vi "GetStateData.vi"(11 "Pod in":T18={"DriveMotorRef"={"DeviceStatus"={"status"=FALSE, "code"=0, "source"=""}, "Type"=enum."PWM", "PWM"={"Controller"=enum."Controller 1", "PWM Channel"=enum."Invalid", "DeadBand"={"Name"="", "maxPositivePwm"=0, "minPositivePwm"=0, "centerPwm"=0, "maxNegativePwm"=0, "minNegativePwm"=0, "angularRange"=0}}, "CAN"={"Device Number"=0, "Control Mode"=enum."Percent VBus", "Semaphore"=refnum, "Max Vout"=12.0, "TalonSRX Control Mode"=enum."Percent VBus"}, "Invert"=FALSE, "TransformRef"=refnum, "InvTransformRef"=refnum}, "TurretMotorRef"={"DeviceStatus"={"status"=FALSE, "code"=0, "source"=""}, "Type"=enum."PWM", "PWM"={"Controller"=enum."Controller 1", "PWM Channel"=enum."Invalid", "DeadBand"={"Name"="", "maxPositivePwm"=0, "minPositivePwm"=0, "centerPwm"=0, "maxNegativePwm"=0, "minNegativePwm"=0, "angularRange"=0}}, "CAN"={"Device Number"=0, "Control Mode"=enum."Percent VBus", "Semaphore"=refnum, "Max Vout"=12.0, "TalonSRX Control Mode"=enum."Percent VBus"}, "Invert"=FALSE, "TransformRef"=refnum, "InvTransformRef"=refnum}, "Turret Encoder"={"AIDeviceRef"={"DevStatus"={"status"=FALSE, "code"=0, "source"=""}, "Controller"=enum."Controller 1", "Analog Channel"=enum."AI 0"}, "Turret Analog Location"=enum."RoboRio"}, "Drive Encoder"={"EncoderDevRef"={"DevStatus"={"status"=FALSE, "code"=0, "source"=""}, "EncoderIndex"=enum."Invalid", "CounterIndex"=enum."Invalid", "DistancePerCount"=1.0, "Decoding Type"=enum."4x"}, "Drive Encoder Location"=enum."RoboRio"}, "Pod position (RCS)"={"X"=0.0, "Y"=0.0, "Z"=0.0}, "Data"={"Drive Motor Output"=0.0, "Turret Motor Output"=0.0, "Wheel RPM"=0.0, "Turret Angle"=0.0, "Turret angle offset"=0.0, "Transmission moment of inertia"=0.0, "Transmission efficiency"=0.0, "Wheel dist / rev"=0.0, "Turret moment of inertia"=0.0, "Inv. turret encoder"=FALSE, "Inv. drive encoder"=FALSE}}) -> (2 "Pod States":T1, 3 "Pod out":T18={"DriveMotorRef"={"DeviceStatus"={"status"=FALSE, "code"=0, "source"=""}, "Type"=enum."PWM", "PWM"={"Controller"=enum."Controller 1", "PWM Channel"=enum."Invalid", "DeadBand"={"Name"="", "maxPositivePwm"=0, "minPositivePwm"=0, "centerPwm"=0, "maxNegativePwm"=0, "minNegativePwm"=0, "angularRange"=0}}, "CAN"={"Device Number"=0, "Control Mode"=enum."Percent VBus", "Semaphore"=refnum, "Max Vout"=12.0, "TalonSRX Control Mode"=enum."Percent VBus"}, "Invert"=FALSE, "TransformRef"=refnum, "InvTransformRef"=refnum}, "TurretMotorRef"={"DeviceStatus"={"status"=FALSE, "code"=0, "source"=""}, "Type"=enum."PWM", "PWM"={"Controller"=enum."Controller 1", "PWM Channel"=enum."Invalid", "DeadBand"={"Name"="", "maxPositivePwm"=0, "minPositivePwm"=0, "centerPwm"=0, "maxNegativePwm"=0, "minNegativePwm"=0, "angularRange"=0}}, "CAN"={"Device Number"=0, "Control Mode"=enum."Percent VBus", "Semaphore"=refnum, "Max Vout"=12.0, "TalonSRX Control Mode"=enum."Percent VBus"}, "Invert"=FALSE, "TransformRef"=refnum, "InvTransformRef"=refnum}, "Turret Encoder"={"AIDeviceRef"={"DevStatus"={"status"=FALSE, "code"=0, "source"=""}, "Controller"=enum."Controller 1", "Analog Channel"=enum."AI 0"}, "Turret Analog Location"=enum."RoboRio"}, "Drive Encoder"={"EncoderDevRef"={"DevStatus"={"status"=FALSE, "code"=0, "source"=""}, "EncoderIndex"=enum."Invalid", "CounterIndex"=enum."Invalid", "DistancePerCount"=1.0, "Decoding Type"=enum."4x"}, "Drive Encoder Location"=enum."RoboRio"}, "Pod position (RCS)"={"X"=0.0, "Y"=0.0, "Z"=0.0}, "Data"={"Drive Motor Output"=0.0, "Turret Motor Output"=0.0, "Wheel RPM"=0.0, "Turret Angle"=0.0, "Turret angle offset"=0.0, "Transmission moment of inertia"=0.0, "Transmission efficiency"=0.0, "Wheel dist / rev"=0.0, "Turret moment of inertia"=0.0, "Inv. turret encoder"=FALSE, "Inv. drive encoder"=FALSE}})   [LabVIEW 2014]
uses:
  <vilib>/Rock Robotics/WPI/MotorControl/WPI_MotorControlDeviceRef.ctl
  <vilib>/Rock Robotics/WPI/MotorControl/WPI_MotorControlType.ctl
  <vilib>/Rock Robotics/SystemInterfaces/Typedef/FPGA_TypedefDigitalModule.ctl
  <vilib>/Rock Robotics/SystemInterfaces/DIO/FPGA_DIOPWMChannel.ctl
  <vilib>/Rock Robotics/WPI/PWM/WPI_PWMDeadband.ctl
  <vilib>/Rock Robotics/WPI/CAN/Jaguar/SubVIs/WPI_CANJaguar_ControlMode.ctl
  <vilib>/Rock Robotics/WPI/CAN/TalonSRX/WPI_CANTalonSRX_APIControlMode.ctl
  <vilib>/Rock Robotics/WPI/PWM/WPI_PWMTransform_ConPane.ctl
  <vilib>/Rock Robotics/WPI/AnalogChannel/WPI_AnalogChannelDevRef.ctl
  <vilib>/Rock Robotics/SystemInterfaces/Typedef/FPGA_TypedefAnalogModule.ctl
  <vilib>/Rock Robotics/SystemInterfaces/AI/FPGA_AIChannel.ctl
  <vilib>/Rock Robotics/WPI/Encoder/WPI_EncoderDevRef.ctl
  <vilib>/Rock Robotics/SystemInterfaces/Encoder/FPGA_EncoderIdx.ctl
  <vilib>/Rock Robotics/SystemInterfaces/Counter/FPGA_CounterCtrSystemIndex.ctl
  <vilib>/Rock Robotics/WPI/Encoder/WPI_EncoderType.ctl
  <vilib>/Rock Robotics/SystemInterfaces/Utilities/FPGA_UtilitiesRead LocalTime.vi
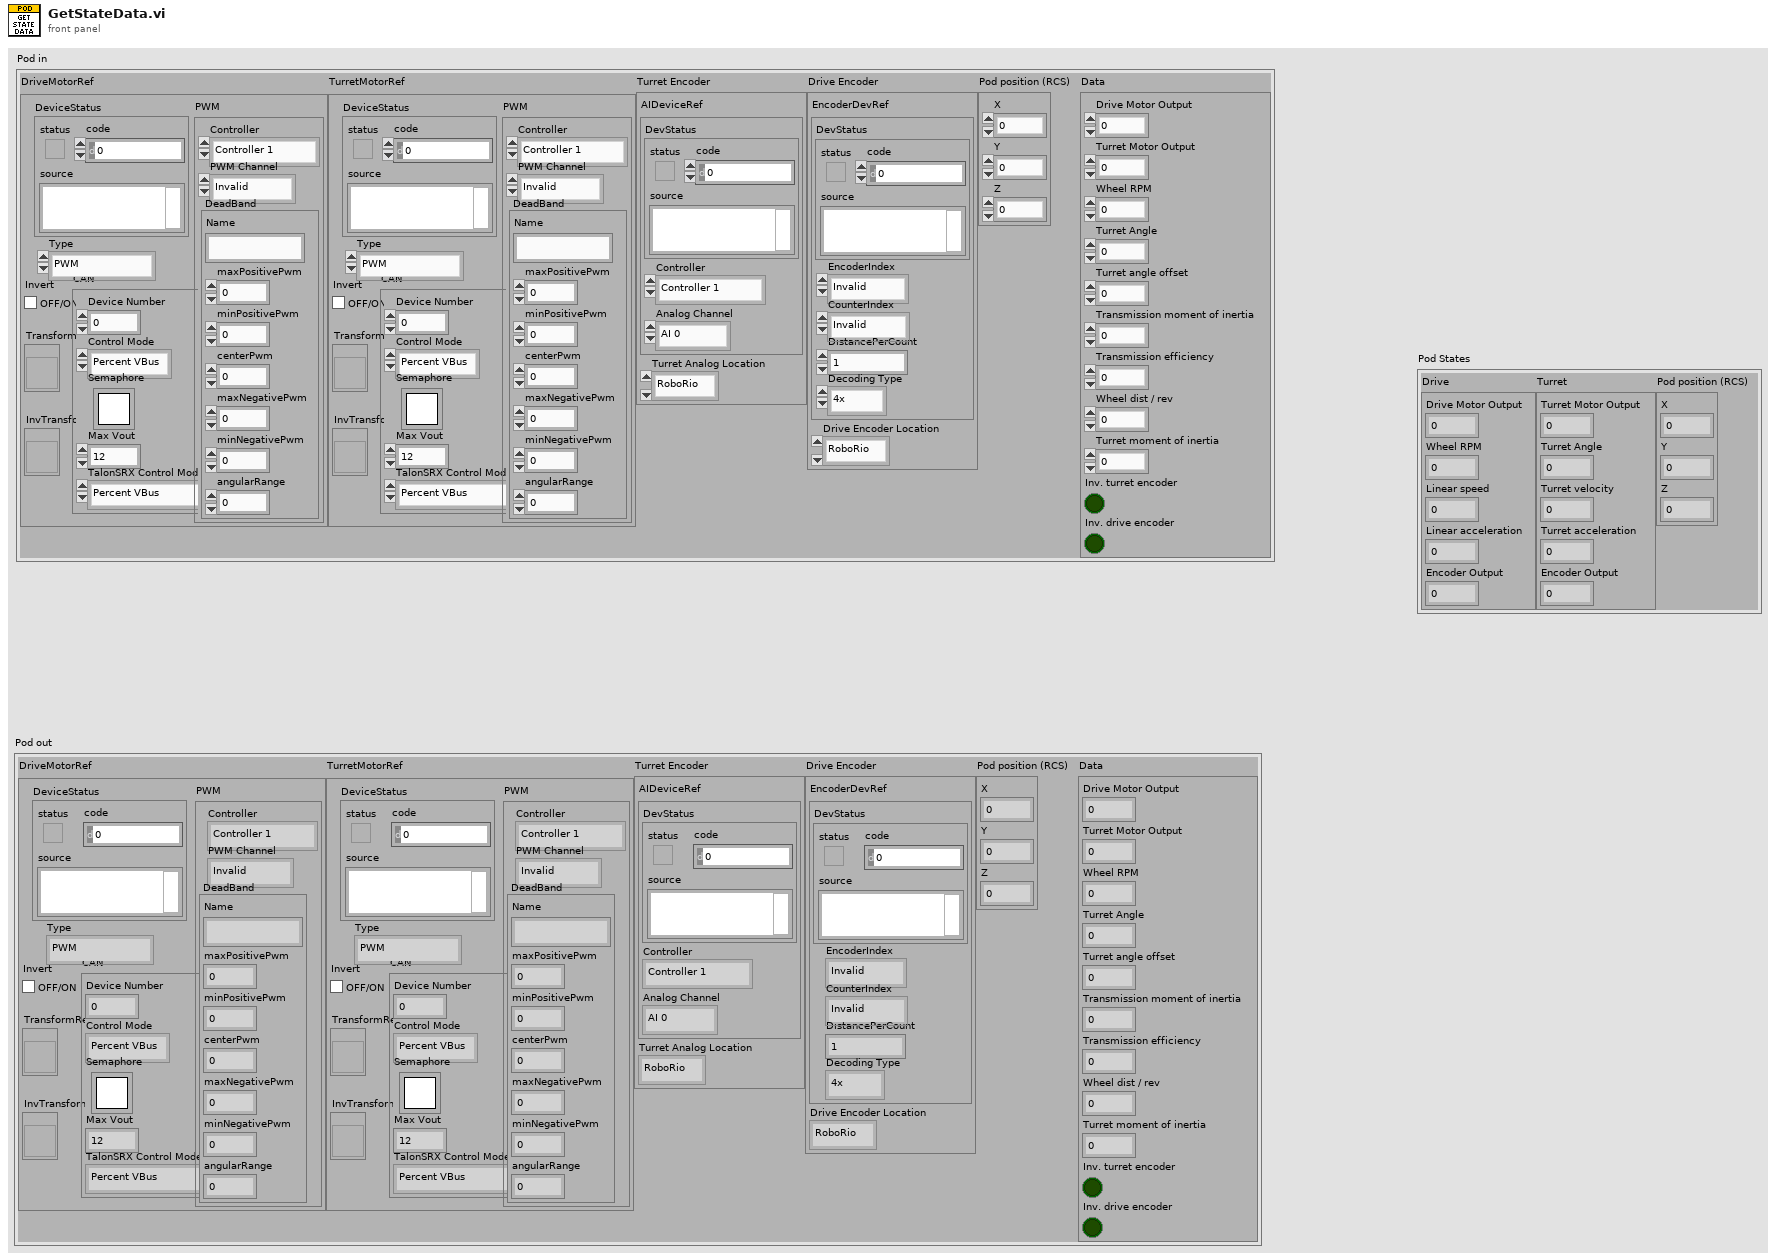
[diagram p1: front panel]
types:
  T1 = cluster{"Drive":cluster{"Drive Motor Output":dbl, "Wheel RPM":dbl, "Linear speed":dbl, "Linear acceleration":dbl, "Encoder Output":dbl}, "Turret":cluster{"Turret Motor Output":dbl, "Turret Angle":dbl, "Turret velocity":dbl, "Turret acceleration":dbl, "Encoder Output":dbl}, "Pod position (RCS)":cluster{"X":dbl, "Y":dbl, "Z":dbl}}
  T2 = typedef "WPI_MotorControlDeviceRef.ctl" = cluster{"DeviceStatus":errorcluster, "Type":T3, "PWM":cluster{"Controller":T4, "PWM Channel":T5, "DeadBand":T6}, "CAN":cluster{"Device Number":u8, "Control Mode":T7, "Semaphore":T8, "Max Vout":dbl, "TalonSRX Control Mode":T9}, "Invert":bool, "TransformRef":T10, "InvTransformRef":T10}
  T3 = typedef "WPI_MotorControlType.ctl" = enum16{"PWM", "CAN", "CANTalonSRX"}
  T4 = typedef "FPGA_TypedefDigitalModule.ctl" = enum16{"Controller 1"}
  T5 = typedef "FPGA_DIOPWMChannel.ctl" = enum8{"PWM 0", "PWM 1", "PWM 2", "PWM 3", "PWM 4", "PWM 5", "PWM 6", "PWM 7", "PWM 8", "PWM 9", "PWM MXP 0", "PWM MXP 1", "PWM MXP 2", "PWM MXP 3", "PWM MXP 4", "PWM MXP 5", "PWM MXP 6", "PWM MXP 7", "PWM MXP 8", "PWM MXP 9", "Invalid"}
  T6 = typedef "WPI_PWMDeadband.ctl" = cluster{"Name":string, "maxPositivePwm":i32, "minPositivePwm":i32, "centerPwm":i32, "maxNegativePwm":i32, "minNegativePwm":i32, "angularRange":u16}
  T7 = typedef "WPI_CANJaguar_ControlMode.ctl" = enum8{"Percent VBus", "Current", "Speed", "Position", "Voltage"}
  T8 = typedef "Semaphore RefNum" = refnum<k1>
  T9 = typedef "WPI_CANTalonSRX_APIControlMode.ctl" = enum8{"Percent VBus", "Speed", "Position", "Slave", "Unchanged / Invalid"}
  T10 = typedef "WPI_PWMTransform_ConPane.ctl" = refnum<vi>
  T11 = typedef "WPI_AnalogChannelDevRef.ctl" = cluster{"DevStatus":errorcluster, "Controller":T12, "Analog Channel":T13}
  T12 = typedef "FPGA_TypedefAnalogModule.ctl" = enum16{"Controller 1"}
  T13 = typedef "FPGA_AIChannel.ctl" = enum8{"AI 0", "AI 1", "AI 2", "AI 3", "AI MXP 0", "AI MXP 1", "AI MXP 2", "AI MXP 3", "Invalid"}
  T14 = typedef "WPI_EncoderDevRef.ctl" = cluster{"DevStatus":errorcluster, "EncoderIndex":T15, "CounterIndex":T16, "DistancePerCount":dbl, "Decoding Type":T17}
  T15 = typedef "FPGA_EncoderIdx.ctl" = enum8{"Enc 0", "Enc 1", "Enc 2", "Enc 3", "Enc 4", "Enc 5", "Enc 6", "Enc 7", "Invalid"}
  T16 = typedef "FPGA_CounterCtrSystemIndex.ctl" = enum8{"Ctr 0", "Ctr 1", "Ctr 2", "Ctr 3", "Ctr 4", "Ctr 5", "Ctr 6", "Ctr 7", "Invalid"}
  T17 = typedef "WPI_EncoderType.ctl" = enum16{"1x", "2x", "4x"}
  T18 = cluster{"DriveMotorRef":T2, "TurretMotorRef":T2, "Turret Encoder":cluster{"AIDeviceRef":T11, "Turret Analog Location":enum16{"RoboRio", "Drive SRX", "Turret SRX"}}, "Drive Encoder":cluster{"EncoderDevRef":T14, "Drive Encoder Location":enum16{"RoboRio", "Drive SRX", "Turret SRX"}}, "Pod position (RCS)":cluster{"X":dbl, "Y":dbl, "Z":dbl}, "Data":cluster{"Drive Motor Output":dbl, "Turret Motor Output":dbl, "Wheel RPM":dbl, "Turret Angle":dbl, "Turret angle offset":dbl, "Transmission moment of inertia":dbl, "Transmission efficiency":dbl, "Wheel dist / rev":dbl, "Turret moment of inertia":dbl, "Inv. turret encoder":bool, "Inv. drive encoder":bool}}
  T19 = typedef "WPI_CANTalonSRX_GlobalStatus.ctl" = cluster{"Applied Throttle":dbl, "Module Enabled":bool, "CAN Error":errorcluster, "Closed Loop Error":dbl, "Forward Limit Switch Closed":bool, "Reverse Limit Switch Closed":bool, "Sensor Position":dbl, "Sensor Velocity":dbl, "Current":dbl, "Sticky Fault - Over Temp":bool, "Sticky Fault - Under Voltage":bool, "Sticky Fault - Forward Limit":bool, "Sticky Fault - Reverse Limit":bool, "Sticky Fault - Forward Soft Limit":bool, "Sticky Fault - Reverse Soft Limit":bool, "Brake is Enabled":bool, "Encoder Position":dbl, "Encoder Velocity":dbl, "Encoder Index Count":dbl, "Encoder A Pin State":bool, "Encoder B Pin State":bool, "Encoder Index Pin State":bool, "Analog In":dbl, "Analog In Velocity":dbl, "Temperature (C)":dbl, "Battery Voltage":dbl}
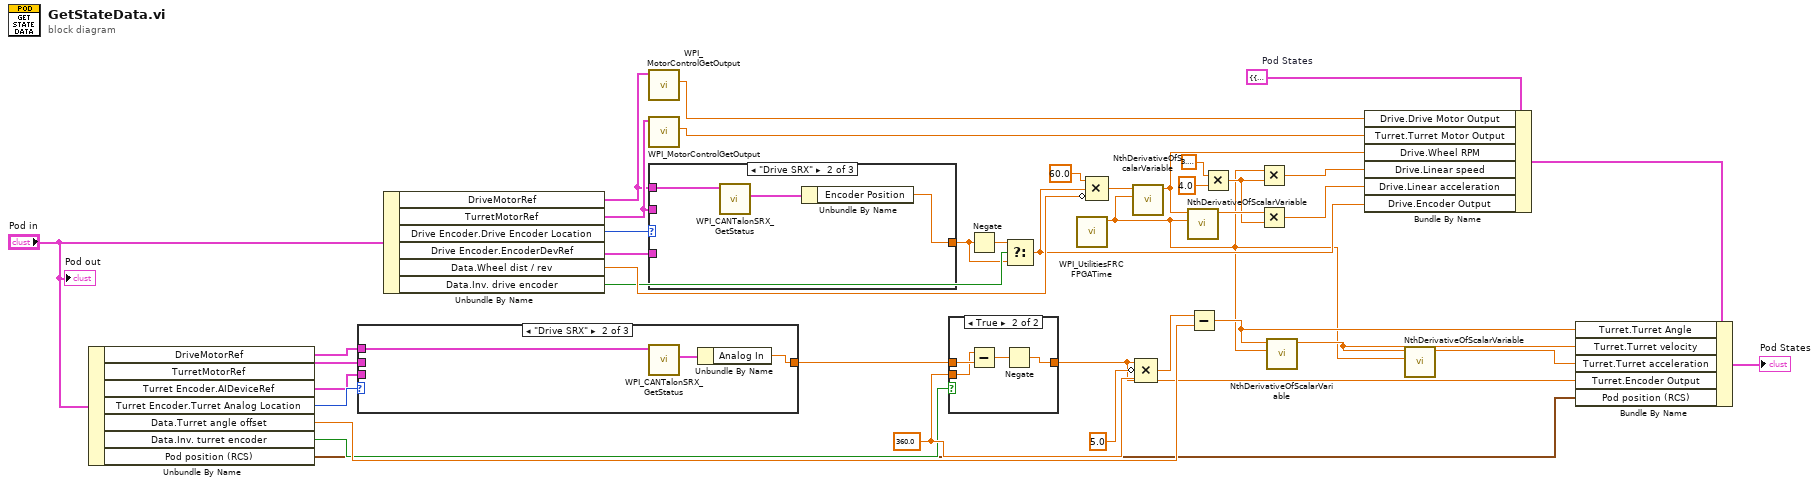
[diagram p0: block diagram]
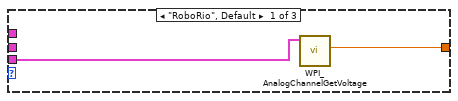
[diagram p3: hidden frame]
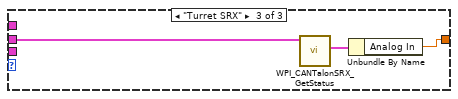
[diagram p4: hidden frame]
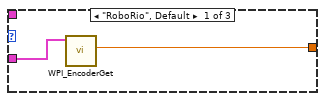
[diagram p5: hidden frame]
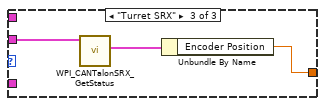
[diagram p6: hidden frame]
diagram:
  w20 = T1 {"Drive"={"Drive Motor Output"=0.0, "Wheel RPM"=0.0, "Linear speed"=0.0, "Linear acceleration"=0.0, "Encoder Output"=0.0}, "Turret"={"Turret Motor Output"=0.0, "Turret Angle"=0.0, "Turret velocity"=0.0, "Turret acceleration"=0.0, "Encoder Output"=0.0}, "Pod position (RCS)"={"X"=0.0, "Y"=0.0, "Z"=0.0}}  # Pod States
  w23 = 360.0 ("value")
  n1 = Unbundle By Name("Pod in") -> ("DriveMotorRef"=w30:T2, "TurretMotorRef"=w31:T2, "Turret Encoder.AIDeviceRef"=w32:T11, "Turret Encoder.Turret Analog Location"=w33:enum16{"RoboRio", "Drive SRX", "Turret SRX"}, "Data.Turret angle offset"=w26:dbl, "Data.Inv. turret encoder"=w22:bool, "Pod position (RCS)"=w12:cluster{"X":dbl, "Y":dbl, "Z":dbl})
  n2 = case shown="\"Drive SRX\"" w33 {
    tunnel: w32 -> [w42 _ _]
    tunnel: w31 -> [_ _ w46]
    tunnel: w30 -> [_ w44 _]
    tunnel: [w41 w43 w47] -> w7
    frame "RoboRio", Default {
      n3 = call <vilib>:"WPI_AnalogChannelGetVoltage.vi"("AIDeviceRef"=w42) -> ("Voltage"=w41:dbl)  [unwired: 8 in, 2 out]
    }
    frame "Drive SRX" {
      n4 = call <vilib>:"WPI_CANTalonSRX_GetStatus.vi"("CAN Talon SRX Ref"=w44) -> ("Talon SRX Status"=w45:T19)  [unwired: 8 in, 2 out]
      n5 = Unbundle By Name(w45) -> ("Analog In"=w43:dbl)
    }
    frame "Turret SRX" {
      n6 = call <vilib>:"WPI_CANTalonSRX_GetStatus.vi"("CAN Talon SRX Ref"=w46) -> ("Talon SRX Status"=w48:T19)  [unwired: 8 in, 2 out]
      n7 = Unbundle By Name(w48) -> ("Analog In"=w47:dbl)
    }
  }
  n8 = Unbundle By Name("Pod in") -> ("DriveMotorRef"=w39:T2, "TurretMotorRef"=w40:T2, "Drive Encoder.Drive Encoder Location"=w38:enum16{"RoboRio", "Drive SRX", "Turret SRX"}, "Drive Encoder.EncoderDevRef"=w37:T14, "Data.Wheel dist / rev"=w36:dbl, "Data.Inv. drive encoder"=w24:bool)
  n9 = call <vilib>:"WPI_MotorControlGetOutput.vi"("MotorControlDevRef"=w39) -> ("Output"=w34:dbl)  [unwired: 8 in, 2 out]
  n10 = call <vilib>:"WPI_MotorControlGetOutput.vi"("MotorControlDevRef"=w40) -> ("Output"=w35:dbl)  [unwired: 8 in, 2 out]
  n11 = case shown="\"Drive SRX\"" w38 {
    tunnel: w40 -> [_ _ w54]
    tunnel: w39 -> [_ w53 _]
    tunnel: w37 -> [w50 _ _]
    tunnel: [w49 w51 w55] -> w10
    frame "RoboRio", Default {
      n12 = call <vilib>:"WPI_EncoderGet.vi"("EncoderDevRef"=w50) -> ("Distance"=w49:dbl)  [unwired: 5 in, 5 out]
    }
    frame "Drive SRX" {
      n13 = call <vilib>:"WPI_CANTalonSRX_GetStatus.vi"("CAN Talon SRX Ref"=w53) -> ("Talon SRX Status"=w52:T19)  [unwired: 8 in, 2 out]
      n14 = Unbundle By Name(w52) -> ("Encoder Position"=w51:dbl)
    }
    frame "Turret SRX" {
      n15 = call <vilib>:"WPI_CANTalonSRX_GetStatus.vi"("CAN Talon SRX Ref"=w54) -> ("Talon SRX Status"=w56:T19)  [unwired: 8 in, 2 out]
      n16 = Unbundle By Name(w56) -> ("Encoder Position"=w55:dbl)
    }
  }
  n17 = case shown="True" w22 {
    tunnel: w7 -> [w57 w61]
    tunnel: w23 -> [_ w60]
    tunnel: [w57 w58] -> w5
    frame False {
    }
    frame True {
      n18 = Subtract(x=w60, y=w61) -> (x-y=w59:dbl)
      n19 = Negate(x=w59) -> (-x=w58:dbl)
    }
  }
  n20 = Negate(x=w10) -> (-x=w25:dbl)
  n21 = Select(t=w25, s=w24, f=w10) -> (s? t:f=w8:dbl)
  n22 = call <vilib>:"WPI_UtilitiesFRC FPGATime.vi"() -> ("FPGA Time"=w1:dbl)  [unwired: 10 in, 1 out]
  n23 = Compound Arithmetic op=MULTIPLY(60.0 ("value"), w8, invert w36) -> (w9:dbl)
  n24 = call "NthDerivativeOfScalarVariable.vi"("FPGA Timestamp"=w1, "X"=w9) -> ("Nth derivative of X"=w11:dbl)  [unwired: 9 in]
  n25 = Compound Arithmetic op=MULTIPLY(w5, invert 5.0 ("value"), w23) -> (w6:dbl)
  n26 = call "NthDerivativeOfScalarVariable.vi"("FPGA Timestamp"=w1, "X"=w11) -> ("Nth derivative of X"=w17:dbl)  [unwired: 9 in]
  n27 = Subtract(x=w6, y=w26) -> (x-y=w4:dbl)
  n28 = Multiply(x=3.141592653589793, y=4.0) -> (x*y=w16:dbl)
  n29 = Multiply(x=w1, y=w16) -> (x*y=w15:dbl)
  n30 = Multiply(x=w17, y=w16) -> (x*y=w14:dbl)
  n31 = call "NthDerivativeOfScalarVariable.vi"("FPGA Timestamp"=w1, "X"=w4) -> ("Nth derivative of X"=w2:dbl)  [unwired: 9 in]
  n32 = Bundle By Name(cluster=w20, "Drive.Drive Motor Output"=w34, "Turret.Turret Motor Output"=w35, "Drive.Wheel RPM"=w11, "Drive.Linear speed"=w15, "Drive.Linear acceleration"=w14, "Drive.Encoder Output"=w8) -> (w27:T1)
  n33 = call "NthDerivativeOfScalarVariable.vi"("FPGA Timestamp"=w1, "X"=w2) -> ("Nth derivative of X"=w3:dbl)  [unwired: 9 in]
  n34 = Bundle By Name(cluster=w27, "Turret.Turret Angle"=w4, "Turret.Turret velocity"=w2, "Turret.Turret acceleration"=w3, "Turret.Encoder Output"=w5, "Pod position (RCS)"=w12) -> (→"Pod States":T1)
  "Pod out" <- "Pod in"
